vi "CameraSendData.vi"(7 "Action":T1, 8 "error in":errorcluster, 11 "name (unnamed)":string) -> (0 "error out":errorcluster, 3 "notifier out":refnum<notifier>)   [LabVIEW 2013]
doc: "NotifierWrapper stores a notifier and allows the user to perform actions on it.\n-Init: create a new notifier with the given data type and name.\n-Get: return a reference to the notifier."
uses:
  NotifierAction.ctl
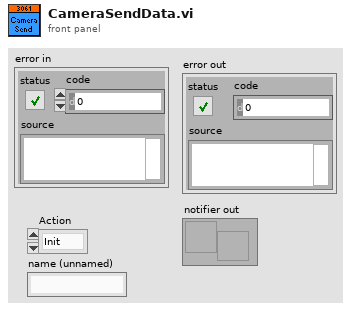
[diagram p1: front panel]
types:
  T1 = typedef "NotifierAction.ctl" = enum16{"Init", "Get"}
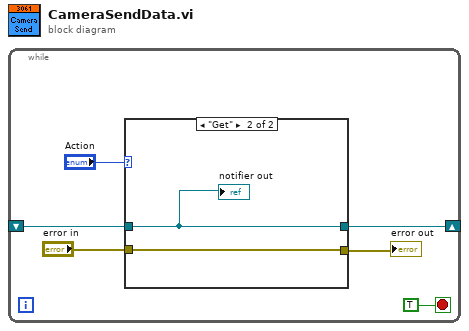
[diagram p0: block diagram]
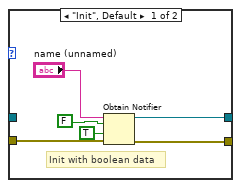
[diagram p2: hidden frame]
diagram:
  n1 = while {
    shift-right: [w2] -> _
    shift-left: _ -> [w1]
    stop <- TRUE stop-if-true
    n2 = case shown="\"Get\"" "Action" {
      tunnel: "error in" -> [w12 w13]
      tunnel: [w10 w13] -> w3
      tunnel: [w9 w14] -> w2
      tunnel: w1 -> [_ w14]
      frame "Init", Default {
        # "Init with boolean data"
        n3 = Obtain Notifier(name (unnamed)="name (unnamed)", notification data type=FALSE, create if not found? (T)=TRUE, error in (no error)=w12) -> (notifier out=w9:refnum<notifier>, error out=w10:errorcluster)  [unwired: 1 out]
      }
      frame "Get" {
        "notifier out" <- w14
      }
    }
    "error out" <- w3
  }
